vi "restFetchStates.vi"(8 "error in (no error)":errorcluster, 11 "JSON String":string) -> (0 "error out":errorcluster, 3 "states":T1(array[cluster]))   [LabVIEW 2018, in "HASS-LV-WS_integration.lvlib"]
uses:
  HASS-LV-WS_integration.lvlib
  <vilib>/addons/_JKI.lib/Serialization/JSON/JKI JSON Serialization.lvlib
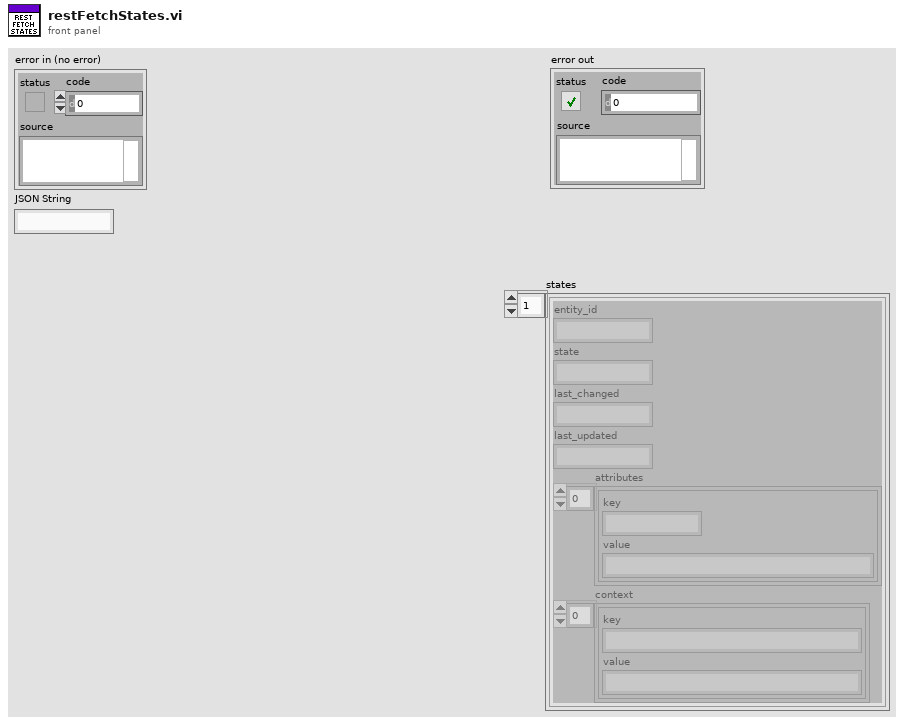
[diagram p1: front panel]
types:
  T1 = cluster{"entity_id":string, "state":string, "last_changed":string, "last_updated":string, "attributes":cluster{"key":string, "value":string}[], "context":cluster{"key":string, "value":string}[]}[]
  T2 = cluster{"entity_id":string, "state":string, "last_changed":string, "last_updated":string, "attributes":cluster{"key":string, "value":string}[], "context":cluster{"key":string, "value":string}[]}
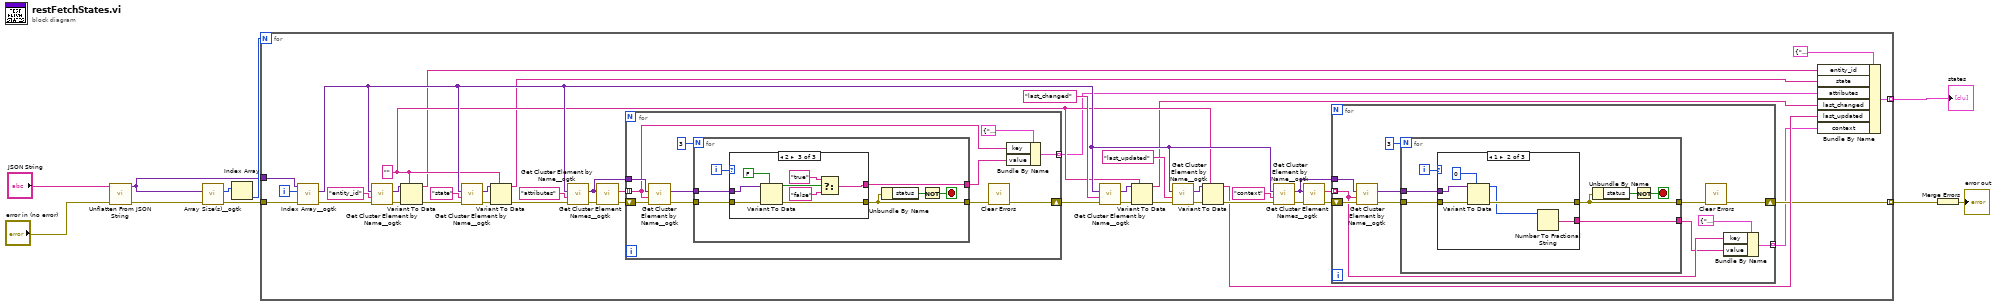
[diagram p0: block diagram]
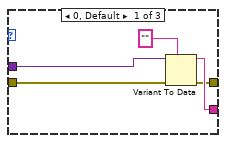
[diagram p2: hidden frame]
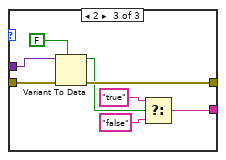
[diagram p3: hidden frame]
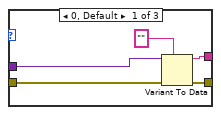
[diagram p4: hidden frame]
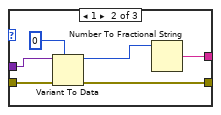
[diagram p5: hidden frame]
diagram:
  n1 = call <vilib>:"Unflatten From JSON String.vi"("error in (no error)"="error in (no error)", "JSON String"="JSON String") -> ("error out"=w3:errorcluster, "Variant"=w4:variant)  [unwired: 8 in]
  n2 = call <userlib>:"Array Size(s)__ogtk.vi"("error in (no error)"=w3, "Array"=w4) -> ("error out"=w7:errorcluster, "Size(s)"=w10:u32[])  [unwired: 7 in, 1 out]
  n3 = Index Array(array=w10) -> (element=w9:u32)  [unwired: 1 in]
  n4 = for {
    N: w9 -> [_]
    tunnel: w4 -> [w52]
    tunnel: [w24] -> w8 mode=indexing
    tunnel: [w14] -> w6 mode=indexing
    tunnel: w7 -> [w11]
    i -> [w51]
    w30 = ""
    n5 = call <userlib>:"Index Array__ogtk.vi"("error in (no error)"=w11, "Index (1D)"=w51, "MultiD Array"=w52) -> ("error out"=w44:errorcluster, "Array Element"=w43:variant)  [unwired: 7 in]
    n6 = call <userlib>:"Get Cluster Element by Name__ogtk.vi"("error in (no error)"=w44, "Element Name"="entity_id", "Cluster"=w43) -> ("error out"=w42:errorcluster, "VElement"=w34:variant)  [unwired: 6 in, 1 out]
    n7 = Variant To Data(error in=w42, type=w30, Variant=w34) -> (data=w28:string, error out=w41:errorcluster)
    n8 = call <userlib>:"Get Cluster Element by Name__ogtk.vi"("error in (no error)"=w41, "Element Name"="state", "Cluster"=w43) -> ("error out"=w40:errorcluster, "VElement"=w33:variant)  [unwired: 6 in, 1 out]
    n9 = Variant To Data(error in=w40, type=w30, Variant=w33) -> (data=w27:string, error out=w39:errorcluster)
    n10 = call <userlib>:"Get Cluster Element by Name__ogtk.vi"("error in (no error)"=w39, "Element Name"="attributes", "Cluster"=w43) -> ("error out"=w21:errorcluster, "VElement"=w23:variant)  [unwired: 6 in, 1 out]
    n11 = call <userlib>:"Get Cluster Element Names__ogtk.vi"("error in (no error)"=w21, "Cluster"=w23) -> ("error out"=w20:errorcluster, "Element Names"=w22:string[])  [unwired: 8 in]
    n12 = for {
      tunnel: w23 -> [w100]
      tunnel: w22 -> [w95] mode=indexing
      shift-right: [w90] -> w19
      shift-left: w20 -> [w97]
      tunnel: [w94] -> w18 mode=indexing
      n13 = call <userlib>:"Get Cluster Element by Name__ogtk.vi"("error in (no error)"=w97, "Element Name"=w95, "Cluster"=w100) -> ("error out"=w99:errorcluster, "VElement"=w92:variant)  [unwired: 6 in, 1 out]
      n14 = for {
        N: 3 -> [_]
        tunnel: [w106] -> w93
        tunnel: w92 -> [w105]
        tunnel: w99 -> [w107]
        tunnel: [w103] -> w98
        i -> [w104]
        stop <- w101 stop-if-true
        n15 = case shown="2" w104 {
          tunnel: w107 -> [w108 w118 w126]
          tunnel: [w109 w115 w124] -> w103
          tunnel: [w110 w113 w120] -> w106
          tunnel: w105 -> [w111 w117 w125]
          frame 0, Default {
            n16 = Variant To Data(error in=w108, type="", Variant=w111) -> (data=w110:string, error out=w109:errorcluster)
          }
          frame 1 {
            n17 = Variant To Data(error in=w118, type=0, Variant=w117) -> (data=w114:i32, error out=w115:errorcluster)
            n18 = Number To Fractional String(number=w114) -> (F-format string=w113:string)  [unwired: 3 in]
          }
          frame 2 {
            n19 = Variant To Data(error in=w126, type=FALSE, Variant=w125) -> (data=w122:bool, error out=w124:errorcluster)
            n20 = Select(t="true", s=w122, f="false") -> (s? t:f=w120:string)
          }
        }
        n21 = Unbundle By Name(w103) -> ("status"=w102:bool)
        n22 = Not(x=w102) -> (.not. x?=w101:bool)
      }
      n23 = call <vilib>:"Clear Errors.vi"("error in (no error)"=w98) -> ("error out"=w90:errorcluster)  [unwired: 5 in, 1 out]
      n24 = Bundle By Name(cluster=cluster{"key":string, "value":string} {"key"="", "value"=""}, "key"=w95, "value"=w93) -> (w94:cluster{"key":string, "value":string})
    }
    n25 = call <userlib>:"Get Cluster Element by Name__ogtk.vi"("error in (no error)"=w19, "Element Name"="last_changed", "Cluster"=w43) -> ("error out"=w38:errorcluster, "VElement"=w32:variant)  [unwired: 6 in, 1 out]
    n26 = Variant To Data(error in=w38, type=w30, Variant=w32) -> (data=w26:string, error out=w37:errorcluster)
    n27 = call <userlib>:"Get Cluster Element by Name__ogtk.vi"("error in (no error)"=w37, "Element Name"="last_updated", "Cluster"=w43) -> ("error out"=w36:errorcluster, "VElement"=w31:variant)  [unwired: 6 in, 1 out]
    n28 = Variant To Data(error in=w36, type=w30, Variant=w31) -> (data=w25:string, error out=w35:errorcluster)
    n29 = call <userlib>:"Get Cluster Element by Name__ogtk.vi"("error in (no error)"=w35, "Element Name"="context", "Cluster"=w43) -> ("error out"=w17:errorcluster, "VElement"=w13:variant)  [unwired: 6 in, 1 out]
    n30 = call <userlib>:"Get Cluster Element Names__ogtk.vi"("error in (no error)"=w17, "Cluster"=w13) -> ("error out"=w16:errorcluster, "Element Names"=w15:string[])  [unwired: 8 in]
    n31 = for {
      tunnel: w13 -> [w63]
      tunnel: w15 -> [w60] mode=indexing
      shift-right: [w54] -> w14
      shift-left: w16 -> [w62]
      tunnel: [w59] -> w12 mode=indexing
      n32 = call <userlib>:"Get Cluster Element by Name__ogtk.vi"("error in (no error)"=w62, "Element Name"=w60, "Cluster"=w63) -> ("error out"=w58:errorcluster, "VElement"=w57:variant)  [unwired: 6 in, 1 out]
      n33 = for {
        N: 3 -> [_]
        tunnel: [w69] -> w55
        tunnel: w57 -> [w68]
        tunnel: w58 -> [w70]
        tunnel: [w66] -> w56
        i -> [w67]
        stop <- w64 stop-if-true
        n34 = case shown="1" w67 {
          tunnel: w70 -> [w71 w81 w89]
          tunnel: [w72 w78 w87] -> w66
          tunnel: [w73 w76 w83] -> w69
          tunnel: w68 -> [w74 w80 w88]
          frame 0, Default {
            n35 = Variant To Data(error in=w71, type="", Variant=w74) -> (data=w73:string, error out=w72:errorcluster)
          }
          frame 1 {
            n36 = Variant To Data(error in=w81, type=0, Variant=w80) -> (data=w77:i32, error out=w78:errorcluster)
            n37 = Number To Fractional String(number=w77) -> (F-format string=w76:string)  [unwired: 3 in]
          }
          frame 2 {
            n38 = Variant To Data(error in=w89, type=FALSE, Variant=w88) -> (data=w85:bool, error out=w87:errorcluster)
            n39 = Select(t="true", s=w85, f="false") -> (s? t:f=w83:string)
          }
        }
        n40 = Unbundle By Name(w66) -> ("status"=w65:bool)
        n41 = Not(x=w65) -> (.not. x?=w64:bool)
      }
      n42 = call <vilib>:"Clear Errors.vi"("error in (no error)"=w56) -> ("error out"=w54:errorcluster)  [unwired: 5 in, 1 out]
      n43 = Bundle By Name(cluster=cluster{"key":string, "value":string} {"key"="", "value"=""}, "key"=w60, "value"=w55) -> (w59:cluster{"key":string, "value":string})
    }
    n44 = Bundle By Name(cluster=T2 {"entity_id"="", "state"="", "last_changed"="", "last_updated"="", "attributes"=[], "context"=[]}, "entity_id"=w28, "state"=w27, "attributes"=w18, "last_changed"=w26, "last_updated"=w25, "context"=w12) -> (w24:T2)
  }
  "states" <- w8
  n45 = Merge Errors(w6) -> (→"error out":errorcluster)
